vi "Create Parameter Loader.vi"(8 "Error in":errorcluster caption="Error in (no error)", 11 "Test Template in":refnum<class "Load Defaults.lvclass">) -> (0 "Error out":errorcluster, 3 "Parameter Loader out":refnum<class "Parameter Loader.lvclass">)   [LabVIEW 2015, in "Load Defaults.lvclass"]
uses:
  Load Defaults.lvclass
  Classes/Parameter Loader/Class/Parameter Loader.lvclass
  <vilib>/Cree, Inc/Cree Test Framework/Classes/Base Objects/Base Class/Base Class/Base Class.lvclass
  Test Class/Test Class.lvclass
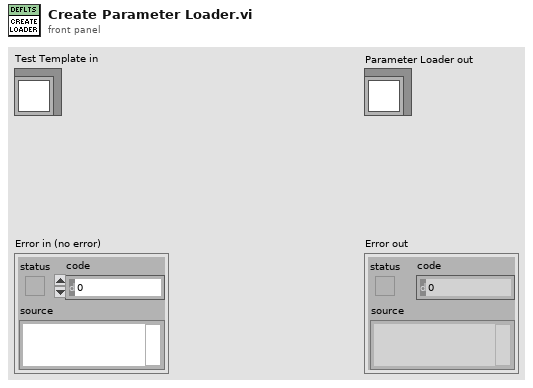
[diagram p1: front panel]
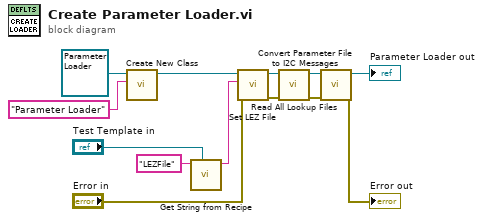
[diagram p0: block diagram]
diagram:
  n1 = call <vilib>:"Create New Class.vi"("Name"="Parameter Loader", "Base Class in"=refnum<class "Parameter Loader.lvclass"> refnum ("Parameter Loader in")) -> ("Base Class out"=w9:refnum<class "Parameter Loader.lvclass">)  [unwired: 8 in, 1 out]
  n2 = call "Get String from Recipe.vi"("Test Class in"="Test Template in", "Name"="LEZFile") -> ("Value"=w3:string)  [unwired: 7 in, 2 out]
  n3 = call "Set LEZ File.vi"("error in (no error)"="Error in", "LEZ File"=w3, "Parameter Loader in"=w9) -> ("error out"=w7:errorcluster, "Parameter Loader out"=w12:refnum<class "Parameter Loader.lvclass">)  [unwired: 7 in]
  n4 = call "Read All Lookup Files.vi"("error in (no error)"=w7, "Parameter Loader in"=w12) -> ("error out"=w6:errorcluster, "Parameter Loader out"=w13:refnum<class "Parameter Loader.lvclass">)  [unwired: 8 in]
  n5 = call "Convert Parameter File to I2C Messages.vi"("error in (no error)"=w6, "Parameter Loader in"=w13) -> ("error out"=→"Error out":errorcluster, "Parameter Loader out"=→"Parameter Loader out":refnum<class "Parameter Loader.lvclass">)  [unwired: 8 in]
